vi "CCD3000 Prepare Acquisition.vi"(4 "Mapping Spectra Settings":T3={"Integration Time"=10.0, "Repetitions"=10, "Mapping Spectra"=TRUE} {"Repetitions" min=1 max=100 step=1; "Integration Time" min=0.5 max=6000.0 step=1.0 format="%.1f"}, 5 "Comm Params":T2={"Comm Interface"=1, "BUS"=0, "Address"=5, "Com Port"=1} {"Comm Interface" items=["RS 232", "GPIB"]}) -> ()   [LabVIEW 2010]
uses:
  Mapping/TypeDefs/Mapping Spectra Params.ctl
  drivers/Horiba Spectrum One 3000V/Lib/CCD_command.llb/Comm Params.ctl
panel:
  out "Region Info Array":T1(array[cluster])=[{"X Origin"=0, "Y Origin"=0, "X Size"=1024, "Y Size"=256, "X Bin"=1, "Y Bin"=1}]
  in  "Imaging Mode":enum16{"1D Spectrum", "2D Image"}(ring)
  out "error out":errorcluster
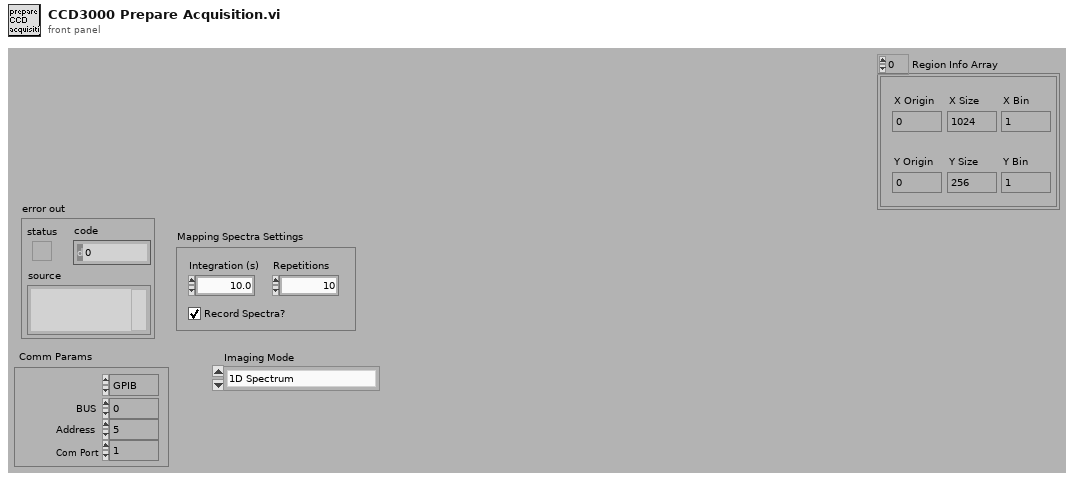
[diagram p1: front panel]
types:
  T1 = cluster{"X Origin":u32, "Y Origin":u32, "X Size":u32, "Y Size":u32, "X Bin":u32, "Y Bin":u32}[]
  T2 = typedef "Comm Params.ctl" = cluster{"Comm Interface":u16, "BUS":i16, "Address":i16, "Com Port":i32}
  T3 = typedef "Mapping Spectra Params.ctl" = cluster{"Integration Time":dbl, "Repetitions":u16, "Mapping Spectra":bool}
  T4 = cluster{"Exposure (ms)":u32, "Interval (ms)":u32, "Flush Count":u32, "Trigger":u16}
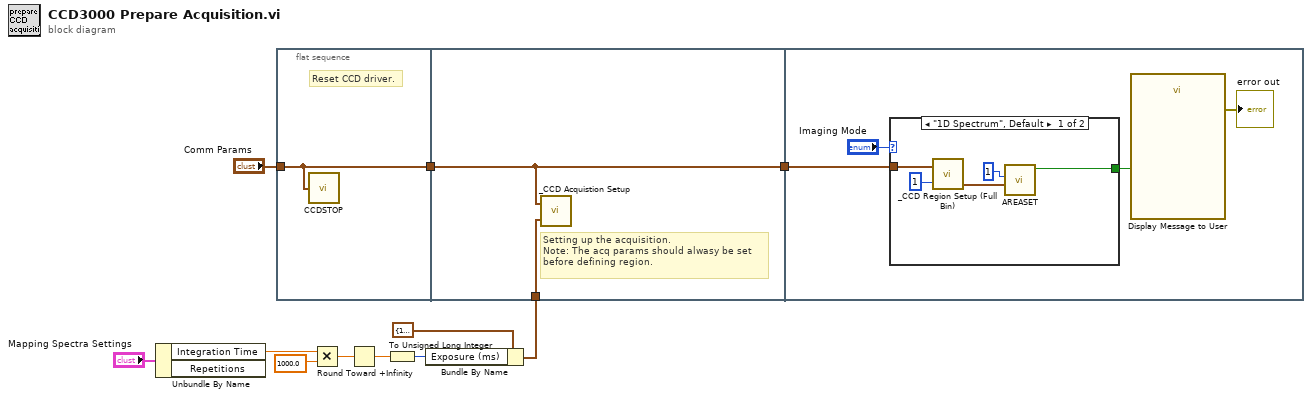
[diagram p0: block diagram]
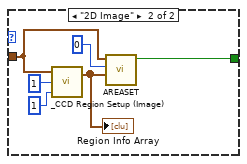
[diagram p2: hidden frame]
diagram:
  n1 = Unbundle By Name("Mapping Spectra Settings") -> ("Integration Time"=w5:dbl)  [unwired: 1 out]
  n2 = flat-sequence {
    tunnel: "Comm Params" -> [w12]
    tunnel: [w12] -> w4
    tunnel: w4 -> [w14]
    tunnel: [w14] -> w3
    tunnel: w1 -> [w13]
    tunnel: w3 -> [w15]
    frame #0 {
      # "Reset CCD driver."
      n3 = call "CCDSTOP.VI"("Comm Params"=w12) -> ()  [unwired: 1 out]
    }
    frame #1 {
      # "Setting up the acquisition.\nNote: The acq params should alwasy be set\nbefore defining region."
      n4 = call "_CCD Acquistion Setup"("Acquisition Param"=w13, "Comm Params"=w14) -> ()  [unwired: 1 out]
    }
    frame #2 {
      n5 = case shown="\"1D Spectrum\", Default" "Imaging Mode" {
        tunnel: [w21 w28] -> w17
        tunnel: w15 -> [w20 w27]
        frame "1D Spectrum", Default {
          n6 = call "_CCD Region Setup (Full Bin)"("Comm Params"=w20, "Number of Regions"=u32 1) -> ("Region Info Array"=w23:T1)  [unwired: 2 out]
          n7 = call "AREASET.VI"("Region Info Array"=w23, "Acquisition Format"=1) -> ("Error"=w21:bool)  [unwired: 6 in]
        }
        frame "2D Image" {
          n8 = call "_CCD Region Setup (Image)"("Y Bin"=u32 1, "X Bin"=u32 1, "Comm Params"=w27) -> ("Region Info Array"=w24:T1)  [unwired: 1 out]
          "Region Info Array" <- w24
          n9 = call "AREASET.VI"("Region Info Array"=w24, "Acquisition Format"=0, "Comm Params"=w27) -> ("Error"=w28:bool)  [unwired: 5 in]
        }
      }
      n10 = call "Display Message to User"("Enable"=w17) -> ("error out"=→"error out":errorcluster)  [unwired: 9 in, 1 out]
    }
  }
  n11 = Multiply(x=w5, y=1000.0) -> (x*y=w9:dbl)
  n12 = Round Toward +Infinity(x=w9) -> (ceil(x): smallest int >= x=w8:dbl)
  n13 = To Unsigned Long Integer(number=w8) -> (unsigned 32bit integer=w7:u32)
  n14 = Bundle By Name(cluster=T4 {"Exposure (ms)"=100, "Interval (ms)"=10, "Flush Count"=1, "Trigger"=0} ("Acquisition Parameters"), "Exposure (ms)"=w7) -> (w1:T4)
